vi "getComPort.vi"(8 "error in (no error)":errorcluster, 11 "Xcite in":refnum<class "Xcite.lvclass">) -> (0 "error out":errorcluster, 2 "com_port":string, 3 "Xcite out":refnum<class "Xcite.lvclass">)   [LabVIEW 2019, in "Xcite.lvclass"]
doc: "Gets the assigned comm port for communication with the XCite device."
uses:
  Xcite.lvclass
  Xcite.lvclass/Xcite.ctl
  etc.xcite/XCite.lvlib
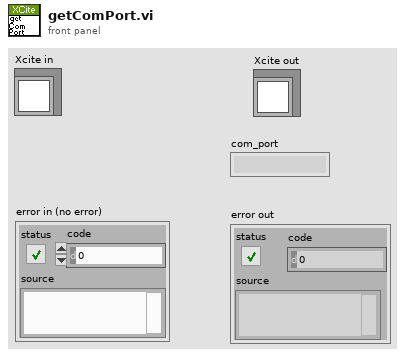
[diagram p1: front panel]
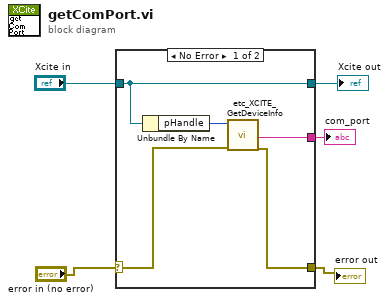
[diagram p0: block diagram]
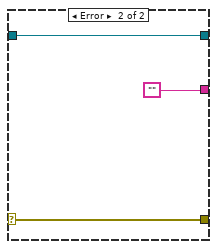
[diagram p2: hidden frame]
diagram:
  n1 = case shown="No Error" "error in (no error)" {
    selector: "error in (no error)" -> [w8 w13]
    tunnel: [w7 w13] -> w4
    tunnel: "Xcite in" -> [w6 w11]
    tunnel: [w9 ""] -> w2
    tunnel: [w6 w11] -> w1
    frame No Error {
      n2 = Unbundle By Name(w6) -> ("pHandle"=w10:u64)
      n3 = call "etc_XCITE_GetDeviceInfo.vi"("h"=w10, "error in (no error)"=w8) -> ("port"=w9:string, "error out"=w7:errorcluster)  [unwired: 12 in, 4 out]
    }
    frame Error {
    }
  }
  "Xcite out" <- w1
  "error out" <- w4
  "com_port" <- w2
